vi "fgv.vi"(7 "Get? (T)":bool=TRUE, 8 "error in (no error)":errorcluster, 10 "Logger Name":string, 11 "RQMHLogger Set":refnum<class "RQMHLogger.lvclass">) -> (0 "error out":errorcluster, 3 "RQMHLogger Get":refnum<class "RQMHLogger.lvclass">)   [LabVIEW 2024, in "RQMHLogSingleton.lvlib"]
uses:
  RQMHLogSingleton.lvlib
  RQMHLogger/RQMHLogger.lvclass
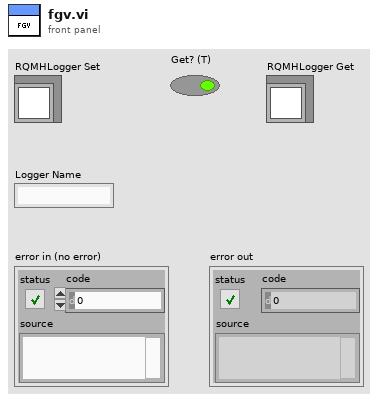
[diagram p1: front panel]
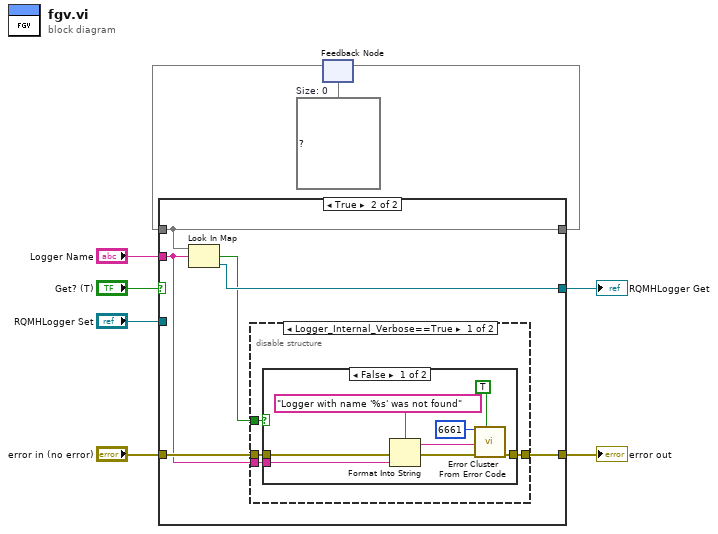
[diagram p0: block diagram]
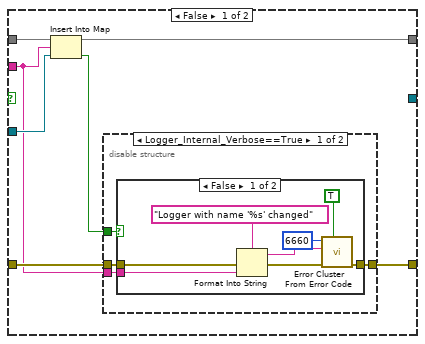
[diagram p2: hidden frame]
diagram:
  w9 = map{string, refnum<class "RQMHLogger.lvclass">} {}  # Size: 0
  n1 = feedback #1(w9) -> (w7:map{string, refnum<class "RQMHLogger.lvclass">})
  n2 = case shown="True" "Get? (T)" {
    tunnel: w7 -> [w16 w36]
    tunnel: [w15 w36] -> w6
    tunnel: "RQMHLogger Set" -> [w14 _]
    tunnel: [_ w35] -> w4
    tunnel: "Logger Name" -> [w10 w31]
    tunnel: "error in (no error)" -> [w13 w33]
    tunnel: [w12 w34] -> w1
    frame False {
      n3 = Insert Into Map(map in=w16, key=w10, value=w14) -> (map out=w15:map{string, refnum<class "RQMHLogger.lvclass">}, value unchanged?=w11:bool)  [unwired: 1 out]
      n4 = disable-structure shown="Logger_Internal_Verbose==True" {
        disable-tunnel: w13 -> [w19 w30]
        disable-tunnel: [w20 w30] -> w12
        disable-tunnel: w11 -> [w18 _]
        disable-tunnel: w10 -> [w17 _]
        frame condition #0 (active) {
          n5 = case shown="False" w18 {
            tunnel: [w28 w29] -> w20
            tunnel: w19 -> [w27 w29]
            tunnel: w17 -> [w23 _]
            frame False {
              n6 = Format Into String(format string="Logger with name '%s' changed", error in=w27, w23) -> (resulting string=w21:string, error out=w25:errorcluster)  [unwired: 1 in]
              n7 = call <vilib>:"Error Cluster From Error Code.vi"("show call chain? (False)"=TRUE, "error in (no error)"=w25, "error message (\"\")"=w21, "error code (0)"=6660) -> ("error out"=w28:errorcluster)  [unwired: 5 in]
            }
            frame True {
            }
          }
        }
        frame condition #1 {
        }
      }
    }
    frame True {
      n8 = Look In Map(map=w36, key=w31) -> (key not found?=w32:bool, value=w35:refnum<class "RQMHLogger.lvclass">)  [unwired: 1 in]
      n9 = disable-structure shown="Logger_Internal_Verbose==True" {
        disable-tunnel: w33 -> [w39 w50]
        disable-tunnel: [w40 w50] -> w34
        disable-tunnel: w32 -> [w38 _]
        disable-tunnel: w31 -> [w37 _]
        frame condition #0 (active) {
          n10 = case shown="False" w38 {
            tunnel: [w48 w49] -> w40
            tunnel: w39 -> [w47 w49]
            tunnel: w37 -> [w43 _]
            frame False {
              n11 = Format Into String(format string="Logger with name '%s' was not found", error in=w47, w43) -> (resulting string=w42:string, error out=w45:errorcluster)  [unwired: 1 in]
              n12 = call <vilib>:"Error Cluster From Error Code.vi"("show call chain? (False)"=TRUE, "error in (no error)"=w45, "error message (\"\")"=w42, "error code (0)"=6661) -> ("error out"=w48:errorcluster)  [unwired: 5 in]
            }
            frame True {
            }
          }
        }
        frame condition #1 {
        }
      }
    }
  }
  "RQMHLogger Get" <- w4
  "error out" <- w1
  n13 = feedback-in #1(w6) -> ()
